vi "CMN_Write_Characterss_To_File.vi"(0 "convert eol? (no:F)":bool, 3 "append to file? (new file:F)":bool, 4 "character string":string, 5 "file path (dialog if empty)":path) -> (1 "error out":errorcluster, 2 "new file path (Not A Path if cancelled)":path)   [LabVIEW 2016]
doc: "Writes a <B>character string</B> to a new byte stream file or appends the string to an existing file. The VI opens or creates the file before writing to it and closes it afterwards."
panel:
  in  "prompt":string="Choose file to write."
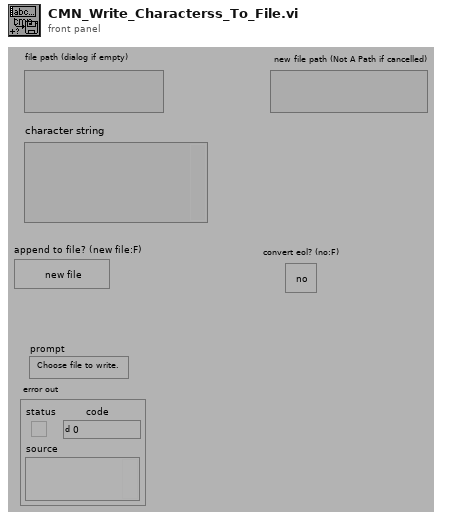
[diagram p1: front panel]
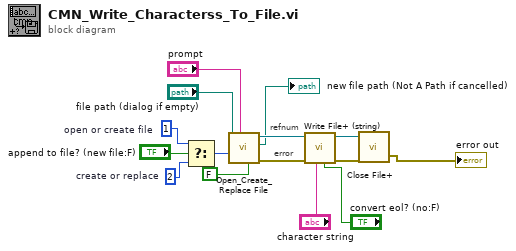
[diagram p0: block diagram]
diagram:
  w7 = i16 2  # create or replace
  w10 = i16 1  # open or create file
  # "error"
  # "refnum"
  n1 = Select(t=w10, s="append to file? (new file:F)", f=w7) -> (s? t:f=w11:i16)
  n2 = call <vilib>:"Open_Create_Replace File.vi"("advisory dialog? (display:T)"=FALSE, "prompt"="prompt", "function (open:0)"=w11, "file path"="file path (dialog if empty)") -> ("error out"=w14:errorcluster, "new file path"=→"new file path (Not A Path if cancelled)":path, "refnum"=w6:refnum<file>)  [unwired: 3 in, 2 out]
  n3 = call <vilib>:"Write File+ (string).vi"("convert eol? (no:F)"="convert eol? (no:F)", "string"="character string", "error in (no error)"=w14, "refnum"=w6) -> ("error out"=w13:errorcluster, "dup refnum"=w12:refnum<file>)  [unwired: 2 in, 2 out]
  n4 = call <vilib>:"Close File+.vi"("error in (no error)"=w13, "refnum"=w12) -> ("error out"=→"error out":errorcluster)  [unwired: 5 out]
